vi "Instructor Write Client.vi"() -> ()   [LabVIEW 2017]
uses:
  <vilib>/OPCUA/controls/Write Status.ctl
  <vilib>/OPCUA/controls/NodeId.ctl
  <vilib>/OPCUA/client/Multiple Write Double Array.vi
  <vilib>/OPCUA/client/Multiple Write Bool Array.vi
  <vilib>/OPCUA/NI OPC UA Client.lvlib
panel:
  in  "Node Status 2":T1 items=["Good"=0, "Uncertain_InitialValue"=1083310080, "Uncertain_LastUsableValue"=1083179008, "Uncertain_SensorNotAccurate"=1083375616, "Uncertain_EngineeringUnitsExceeded"=1083441152, "Bad_NoCommunication"=2150694912, "Bad_NotReadable"=2151284736, "Bad_NotWritable"=2151350272, "Bad_OutOfRange"=2151415808, "Bad_WaitingForInitialData"=2150760448]
  in  "Time Stamp 2":timestamp
  in  "Node Status":T1 items=["Good"=0, "Uncertain_InitialValue"=1083310080, "Uncertain_LastUsableValue"=1083179008, "Uncertain_SensorNotAccurate"=1083375616, "Uncertain_EngineeringUnitsExceeded"=1083441152, "Bad_NoCommunication"=2150694912, "Bad_NotReadable"=2151284736, "Bad_NotWritable"=2151350272, "Bad_OutOfRange"=2151415808, "Bad_WaitingForInitialData"=2150760448]
  in  "Time Stamp":timestamp
  in  "Stop Broadcasting":bool
  in  "Time Stamp":timestamp
  in  "Node Status":T1 items=["Good"=0, "Uncertain_InitialValue"=1083310080, "Uncertain_LastUsableValue"=1083179008, "Uncertain_SensorNotAccurate"=1083375616, "Uncertain_EngineeringUnitsExceeded"=1083441152, "Bad_NoCommunication"=2150694912, "Bad_NotReadable"=2151284736, "Bad_NotWritable"=2151350272, "Bad_OutOfRange"=2151415808, "Bad_WaitingForInitialData"=2150760448]
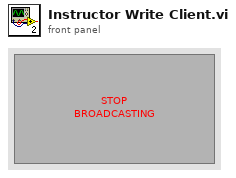
[diagram p1: front panel]
types:
  T1 = typedef "Write Status.ctl" = u32
  T2 = cluster{"message mode":enum16{"None", "Sign", "Sign and Encrypt"}, "security":enum16{"Basic256", "Basic128Rsa15"}}
  T3 = typedef "OPC UA Client Refnum.ctl" = refnum<k21>
  T4 = typedef "NodeId.ctl" = string
  T5 = cluster{"node ID":T4, "value":bool[], "timestamp (current time)":timestamp, "node status":T1}
  T6 = cluster{"node ID":T4, "value":dbl[], "timestamp (current time)":timestamp, "node status":T1}
  T7 = cluster{"node ID":T4, "value":dbl[], "timestamp (current time)":timestamp, "node status":T1}[]
  T8 = cluster{"node ID":T4, "value":bool[], "timestamp (current time)":timestamp, "node status":T1}[]
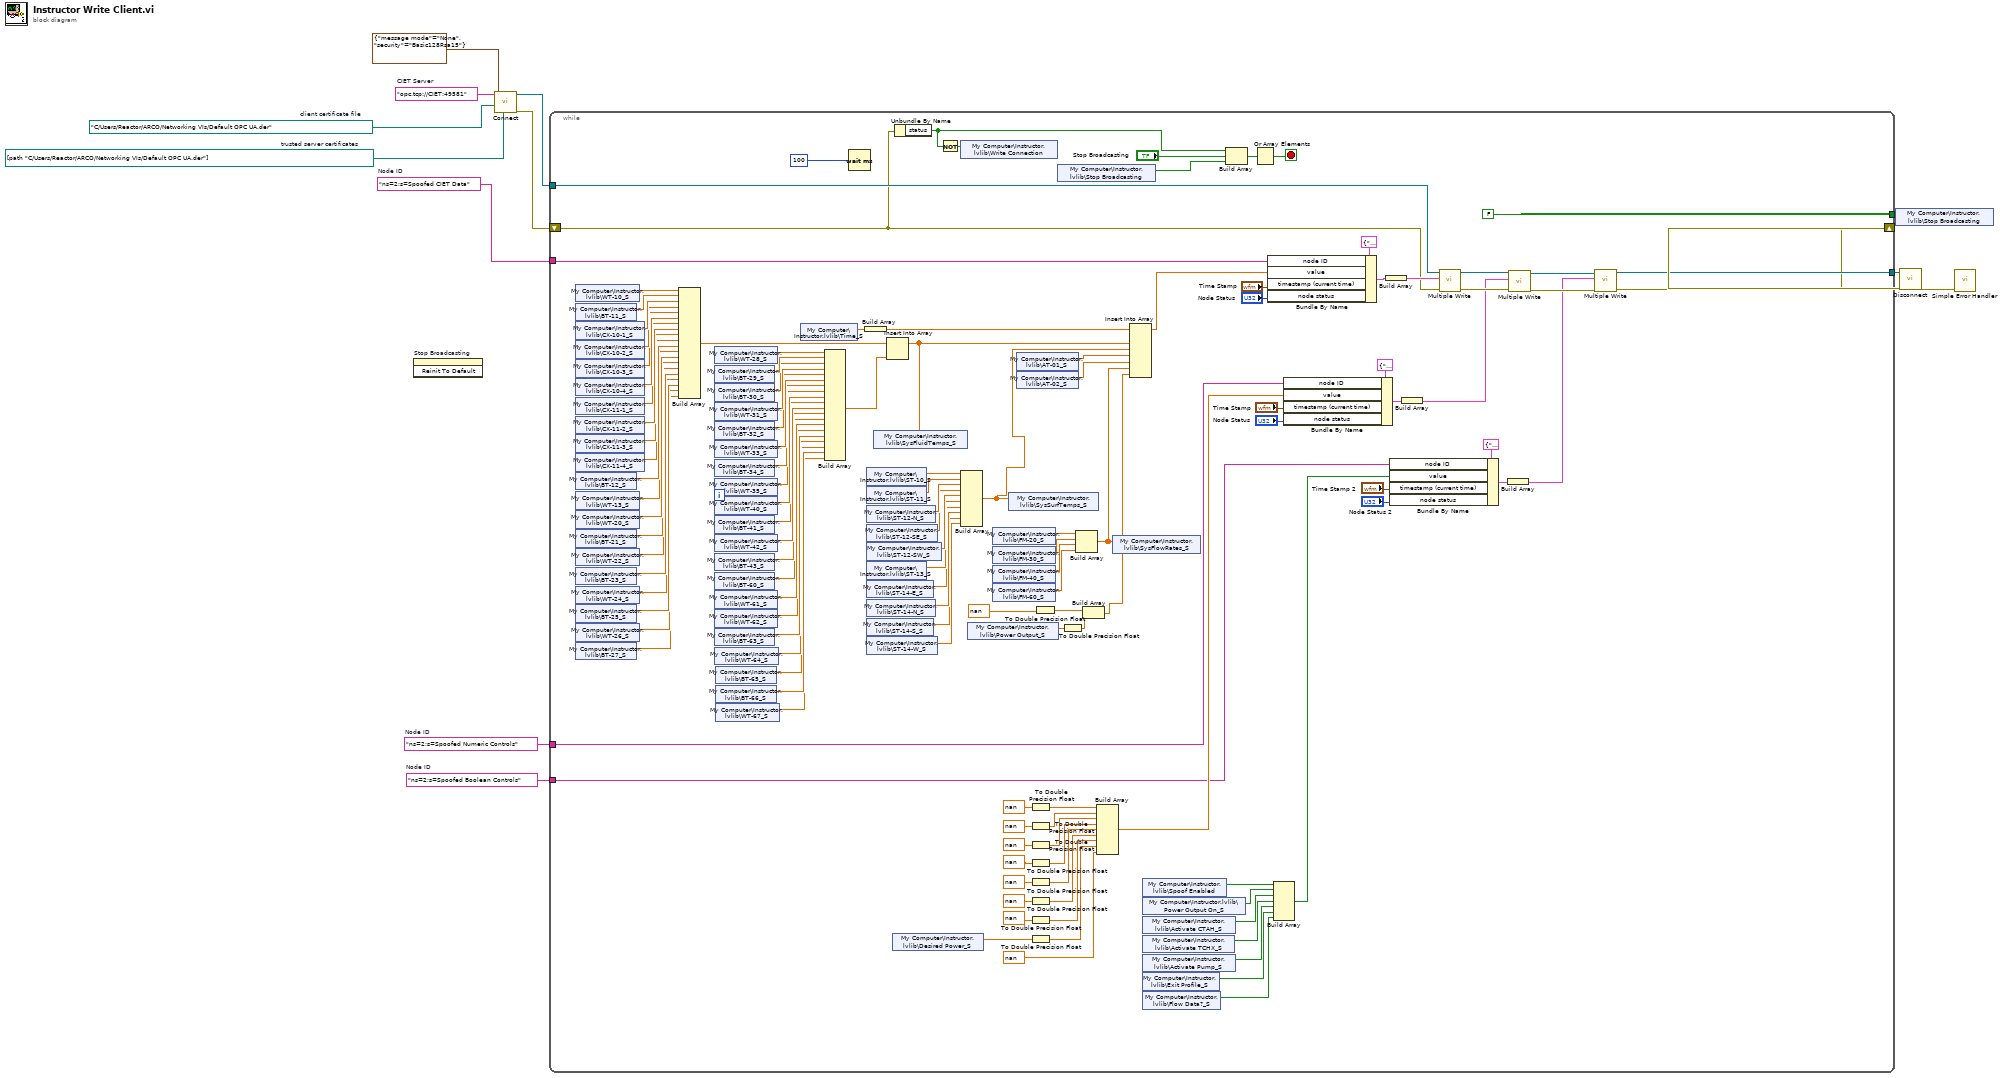
[diagram p0: block diagram]
diagram:
  w1 = "ns=2;s=Spoofed Boolean Controls"  # Node ID
  w3 = "ns=2;s=Spoofed Numeric Controls"  # Node ID
  w8 = path[] [path "C:/Users/Reactor/ARCO/Networking VIs/Default OPC UA.der"]  # trusted server certificates
  w9 = path "C:/Users/Reactor/ARCO/Networking VIs/Default OPC UA.der"  # client certificate file
  w10 = "ns=2;s=Spoofed CIET Data"  # Node ID
  w12 = "opc.tcp://CIET:49581"  # CIET Server
  n1 = invoke on="Stop Broadcasting" class="Bool (strict)" method="Reinit To Default"() -> ()  [unwired: 3 in, 3 out]
  n2 = call <vilib>:"Connect.vi"("trusted server certificates"=w8, "client certificate file"=w9, "security policy"=T2 {"message mode"=enum."None", "security"=enum."Basic128Rsa15"}, "server endpoint URL"=w12) -> ("error out"=w5:errorcluster, "OPC UA client refnum out"=w11:T3)  [unwired: 5 in, 1 out]
  n3 = while {
    tunnel: w10 -> [w141]
    tunnel: w11 -> [w140]
    tunnel: [FALSE] -> w6
    shift-right: [w29] -> w4
    shift-left: w5 -> [w63]
    tunnel: w3 -> [w57]
    tunnel: [w30] -> w2
    tunnel: w1 -> [w28]
    stop <- w69 stop-if-true
    n4 = shared-variable "My Computer\\Instructor.lvlib\\WT-10_S"() -> (w134:sgl)  [unwired: 1 in, 1 out]
    n5 = shared-variable "My Computer\\Instructor.lvlib\\BT-11_S"() -> (w133:sgl)  [unwired: 1 in, 1 out]
    n6 = shared-variable "My Computer\\Instructor.lvlib\\CX-10-1_S"() -> (w132:sgl)  [unwired: 1 in, 1 out]
    n7 = shared-variable "My Computer\\Instructor.lvlib\\CX-10-2_S"() -> (w131:sgl)  [unwired: 1 in, 1 out]
    n8 = shared-variable "My Computer\\Instructor.lvlib\\CX-10-3_S"() -> (w130:sgl)  [unwired: 1 in, 1 out]
    n9 = shared-variable "My Computer\\Instructor.lvlib\\CX-10-4_S"() -> (w129:sgl)  [unwired: 1 in, 1 out]
    n10 = shared-variable "My Computer\\Instructor.lvlib\\CX-11-1_S"() -> (w128:sgl)  [unwired: 1 in, 1 out]
    n11 = shared-variable "My Computer\\Instructor.lvlib\\CX-11-2_S"() -> (w127:sgl)  [unwired: 1 in, 1 out]
    n12 = shared-variable "My Computer\\Instructor.lvlib\\CX-11-3_S"() -> (w126:sgl)  [unwired: 1 in, 1 out]
    n13 = shared-variable "My Computer\\Instructor.lvlib\\CX-11-4_S"() -> (w125:sgl)  [unwired: 1 in, 1 out]
    n14 = shared-variable "My Computer\\Instructor.lvlib\\BT-12_S"() -> (w124:sgl)  [unwired: 1 in, 1 out]
    n15 = shared-variable "My Computer\\Instructor.lvlib\\WT-13_S"() -> (w123:sgl)  [unwired: 1 in, 1 out]
    n16 = shared-variable "My Computer\\Instructor.lvlib\\WT-20_S"() -> (w122:sgl)  [unwired: 1 in, 1 out]
    n17 = shared-variable "My Computer\\Instructor.lvlib\\BT-21_S"() -> (w121:sgl)  [unwired: 1 in, 1 out]
    n18 = shared-variable "My Computer\\Instructor.lvlib\\WT-22_S"() -> (w120:sgl)  [unwired: 1 in, 1 out]
    n19 = shared-variable "My Computer\\Instructor.lvlib\\BT-23_S"() -> (w119:sgl)  [unwired: 1 in, 1 out]
    n20 = shared-variable "My Computer\\Instructor.lvlib\\WT-24_S"() -> (w118:sgl)  [unwired: 1 in, 1 out]
    n21 = shared-variable "My Computer\\Instructor.lvlib\\BT-25_S"() -> (w117:sgl)  [unwired: 1 in, 1 out]
    n22 = shared-variable "My Computer\\Instructor.lvlib\\WT-26_S"() -> (w116:sgl)  [unwired: 1 in, 1 out]
    n23 = shared-variable "My Computer\\Instructor.lvlib\\BT-27_S"() -> (w115:sgl)  [unwired: 1 in, 1 out]
    n24 = Build Array(w134, w133, w132, w131, w130, w129, w128, w127, w126, w125, w124, w123, w122, w121, w120, w119, w118, w117, w116, w115) -> (w93:sgl[])
    n25 = shared-variable "My Computer\\Instructor.lvlib\\WT-28_S"() -> (w114:sgl)  [unwired: 1 in, 1 out]
    n26 = shared-variable "My Computer\\Instructor.lvlib\\BT-29_S"() -> (w113:sgl)  [unwired: 1 in, 1 out]
    n27 = shared-variable "My Computer\\Instructor.lvlib\\BT-30_S"() -> (w112:sgl)  [unwired: 1 in, 1 out]
    n28 = shared-variable "My Computer\\Instructor.lvlib\\WT-31_S"() -> (w111:sgl)  [unwired: 1 in, 1 out]
    n29 = shared-variable "My Computer\\Instructor.lvlib\\BT-32_S"() -> (w110:sgl)  [unwired: 1 in, 1 out]
    n30 = shared-variable "My Computer\\Instructor.lvlib\\WT-33_S"() -> (w109:sgl)  [unwired: 1 in, 1 out]
    n31 = shared-variable "My Computer\\Instructor.lvlib\\BT-34_S"() -> (w108:sgl)  [unwired: 1 in, 1 out]
    n32 = shared-variable "My Computer\\Instructor.lvlib\\WT-35_S"() -> (w107:sgl)  [unwired: 1 in, 1 out]
    n33 = shared-variable "My Computer\\Instructor.lvlib\\WT-40_S"() -> (w106:sgl)  [unwired: 1 in, 1 out]
    n34 = shared-variable "My Computer\\Instructor.lvlib\\BT-41_S"() -> (w105:sgl)  [unwired: 1 in, 1 out]
    n35 = shared-variable "My Computer\\Instructor.lvlib\\WT-42_S"() -> (w104:sgl)  [unwired: 1 in, 1 out]
    n36 = shared-variable "My Computer\\Instructor.lvlib\\BT-43_S"() -> (w103:sgl)  [unwired: 1 in, 1 out]
    n37 = shared-variable "My Computer\\Instructor.lvlib\\BT-60_S"() -> (w102:sgl)  [unwired: 1 in, 1 out]
    n38 = shared-variable "My Computer\\Instructor.lvlib\\WT-61_S"() -> (w101:sgl)  [unwired: 1 in, 1 out]
    n39 = shared-variable "My Computer\\Instructor.lvlib\\WT-62_S"() -> (w100:sgl)  [unwired: 1 in, 1 out]
    n40 = shared-variable "My Computer\\Instructor.lvlib\\BT-63_S"() -> (w99:sgl)  [unwired: 1 in, 1 out]
    n41 = shared-variable "My Computer\\Instructor.lvlib\\WT-64_S"() -> (w98:sgl)  [unwired: 1 in, 1 out]
    n42 = shared-variable "My Computer\\Instructor.lvlib\\BT-65_S"() -> (w97:sgl)  [unwired: 1 in, 1 out]
    n43 = shared-variable "My Computer\\Instructor.lvlib\\BT-66_S"() -> (w96:sgl)  [unwired: 1 in, 1 out]
    n44 = shared-variable "My Computer\\Instructor.lvlib\\WT-67_S"() -> (w95:sgl)  [unwired: 1 in, 1 out]
    n45 = shared-variable "My Computer\\Instructor.lvlib\\Time_S"() -> (w82:sgl)  [unwired: 1 in, 1 out]
    n46 = Build Array(w114, w113, w112, w111, w110, w109, w108, w107, w106, w105, w104, w103, w102, w101, w100, w99, w98, w97, w96, w95) -> (w94:sgl[])
    n47 = Wait (ms)(milliseconds to wait=u32 100) -> ()  [unwired: 1 out]
    n48 = Build Array(w82) -> (w73:sgl[])
    n49 = shared-variable "My Computer\\Instructor.lvlib\\ST-10_S"() -> (w92:sgl)  [unwired: 1 in, 1 out]
    n50 = shared-variable "My Computer\\Instructor.lvlib\\ST-11_S"() -> (w91:sgl)  [unwired: 1 in, 1 out]
    n51 = shared-variable "My Computer\\Instructor.lvlib\\ST-12-N_S"() -> (w90:sgl)  [unwired: 1 in, 1 out]
    n52 = shared-variable "My Computer\\Instructor.lvlib\\ST-12-SE_S"() -> (w89:sgl)  [unwired: 1 in, 1 out]
    n53 = shared-variable "My Computer\\Instructor.lvlib\\ST-12-SW_S"() -> (w88:sgl)  [unwired: 1 in, 1 out]
    n54 = shared-variable "My Computer\\Instructor.lvlib\\ST-13_S"() -> (w87:sgl)  [unwired: 1 in, 1 out]
    n55 = shared-variable "My Computer\\Instructor.lvlib\\ST-14-E_S"() -> (w86:sgl)  [unwired: 1 in, 1 out]
    n56 = shared-variable "My Computer\\Instructor.lvlib\\ST-14-N_S"() -> (w85:sgl)  [unwired: 1 in, 1 out]
    n57 = shared-variable "My Computer\\Instructor.lvlib\\ST-14-S_S"() -> (w84:sgl)  [unwired: 1 in, 1 out]
    n58 = shared-variable "My Computer\\Instructor.lvlib\\ST-14-W_S"() -> (w83:sgl)  [unwired: 1 in, 1 out]
    n59 = Insert Into Array(array=w93, new element=w94) -> (w81:sgl[])  [unwired: 1 in]
    n60 = shared-variable "My Computer\\Instructor.lvlib\\SysFluidTemps_S"(w81) -> ()  [unwired: 1 in, 1 out]
    n61 = shared-variable "My Computer\\Instructor.lvlib\\Desired Power_S"() -> (w50:sgl)  [unwired: 1 in, 1 out]
    n62 = Unbundle By Name(w63) -> ("status"=w65:bool)
    n63 = Not(x=w65) -> (.not. x?=w64:bool)
    n64 = shared-variable "My Computer\\Instructor.lvlib\\Write Connection"(w64) -> ()  [unwired: 1 in, 1 out]
    n65 = Build Array(w92, w91, w90, w89, w88, w87, w86, w85, w84, w83) -> (w72:sgl[])
    n66 = shared-variable "My Computer\\Instructor.lvlib\\Power Output_S"() -> (w17:sgl)  [unwired: 1 in, 1 out]
    n67 = shared-variable "My Computer\\Instructor.lvlib\\FM-20_S"() -> (w78:sgl)  [unwired: 1 in, 1 out]
    n68 = shared-variable "My Computer\\Instructor.lvlib\\FM-30_S"() -> (w77:sgl)  [unwired: 1 in, 1 out]
    n69 = shared-variable "My Computer\\Instructor.lvlib\\FM-40_S"() -> (w76:sgl)  [unwired: 1 in, 1 out]
    n70 = shared-variable "My Computer\\Instructor.lvlib\\FM-60_S"() -> (w75:sgl)  [unwired: 1 in, 1 out]
    n71 = shared-variable "My Computer\\Instructor.lvlib\\SysSurfTemps_S"(w72) -> ()  [unwired: 1 in, 1 out]
    n72 = shared-variable "My Computer\\Instructor.lvlib\\AT-01_S"() -> (w80:sgl)  [unwired: 1 in, 1 out]
    n73 = shared-variable "My Computer\\Instructor.lvlib\\AT-02_S"() -> (w79:sgl)  [unwired: 1 in, 1 out]
    n74 = To Double Precision Float(number=nan) -> (double precision float=w54:dbl)
    n75 = To Double Precision Float(number=nan) -> (double precision float=w53:dbl)
    n76 = To Double Precision Float(number=nan) -> (double precision float=w52:dbl)
    n77 = To Double Precision Float(number=nan) -> (double precision float=w51:dbl)
    n78 = To Double Precision Float(number=nan) -> (double precision float=w49:dbl)
    n79 = To Double Precision Float(number=nan) -> (double precision float=w48:dbl)
    n80 = To Double Precision Float(number=nan) -> (double precision float=w47:dbl)
    n81 = To Double Precision Float(number=w50) -> (double precision float=w46:dbl)
    n82 = To Double Precision Float(number=nan) -> (double precision float=w16:dbl)
    n83 = shared-variable "My Computer\\Instructor.lvlib\\Stop Broadcasting"() -> (w67:bool)  [unwired: 1 in, 1 out]
    n84 = To Double Precision Float(number=w17) -> (double precision float=w15:dbl)
    n85 = Build Array(w78, w77, w76, w75) -> (w74:sgl[])
    n86 = Build Array(w16, w15) -> (w14:dbl[])
    n87 = Build Array(w54, w53, w52, w51, w49, w48, w47, w46, nan ("number")) -> (w45:dbl[])
    n88 = shared-variable "My Computer\\Instructor.lvlib\\SysFlowRates_S"(w74) -> ()  [unwired: 1 in, 1 out]
    n89 = Insert Into Array(array=w73, new element #1=w81, new element #2=w72, new element #3=w80, new element #4=w79, new element #5=w74, new element #6=w14) -> (w71:sgl[])  [unwired: 1 in]
    n90 = shared-variable "My Computer\\Instructor.lvlib\\Spoof Enabled"() -> (w26:bool)  [unwired: 1 in, 1 out]
    n91 = shared-variable "My Computer\\Instructor.lvlib\\Power Output On_S"() -> (w25:bool)  [unwired: 1 in, 1 out]
    n92 = shared-variable "My Computer\\Instructor.lvlib\\Activate CTAH_S"() -> (w24:bool)  [unwired: 1 in, 1 out]
    n93 = shared-variable "My Computer\\Instructor.lvlib\\Activate TCHX_S"() -> (w23:bool)  [unwired: 1 in, 1 out]
    n94 = shared-variable "My Computer\\Instructor.lvlib\\Activate Pump_S"() -> (w22:bool)  [unwired: 1 in, 1 out]
    n95 = shared-variable "My Computer\\Instructor.lvlib\\Exit Profile_S"() -> (w21:bool)  [unwired: 1 in, 1 out]
    n96 = shared-variable "My Computer\\Instructor.lvlib\\Flow Data?_S"() -> (w20:bool)  [unwired: 1 in, 1 out]
    n97 = Build Array(w65, "Stop Broadcasting", w67) -> (w68:bool[])
    n98 = Or Array Elements(Boolean array=w68) -> (logical OR=w69:bool)
    n99 = Bundle By Name(cluster=T6 {"node ID"="", "value"=[], "timestamp (current time)"=timestamp(0 s since 1904-01-01), "node status"=0} ("request"), "node ID"=w141, "value"=w71, "timestamp (current time)"="Time Stamp", "node status"="Node Status") -> (w136:T6)
    n100 = Build Array(w26, w25, w24, w23, w22, w21, w20) -> (w27:bool[])
    n101 = Bundle By Name(cluster=T6 {"node ID"="", "value"=[], "timestamp (current time)"=timestamp(0 s since 1904-01-01), "node status"=0} ("request"), "node ID"=w57, "value"=w45, "timestamp (current time)"="Time Stamp", "node status"="Node Status") -> (w60:T6)
    n102 = Build Array(w136) -> (w135:T7)
    n103 = Bundle By Name(cluster=T5 {"node ID"="", "value"=[], "timestamp (current time)"=timestamp(0 s since 1904-01-01), "node status"=0} ("request"), "node ID"=w28, "value"=w27, "timestamp (current time)"="Time Stamp 2", "node status"="Node Status 2") -> (w36:T5)
    n104 = Build Array(w60) -> (w59:T7)
    n105 = call-poly <vilib>:"Multiple Write.vi"("error in (no error)"=w63, "requests"=w135, "OPC UA client refnum in"=w140) -> ("error out"=w61:errorcluster, "OPC UA client refnum out"=w62:T3)  [unwired: 5 in, 2 out]
    n106 = Build Array(w36) -> (w19:T8)
    n107 = call-poly <vilib>:"Multiple Write.vi"("error in (no error)"=w61, "requests"=w59, "OPC UA client refnum in"=w62) -> ("error out"=w31:errorcluster, "OPC UA client refnum out"=w32:T3)  [unwired: 5 in, 2 out]
    n108 = call-poly <vilib>:"Multiple Write.vi"("error in (no error)"=w31, "requests"=w19, "OPC UA client refnum in"=w32) -> ("error out"=w29:errorcluster, "OPC UA client refnum out"=w30:T3)  [unwired: 5 in, 2 out]
  }
  n109 = shared-variable "My Computer\\Instructor.lvlib\\Stop Broadcasting"(w6) -> ()  [unwired: 1 in, 1 out]
  n110 = call <vilib>:"Disconnect.vi"("error in (no error)"=w4, "OPC UA client refnum in"=w2) -> ("error out"=w13:errorcluster)  [unwired: 9 in]
  n111 = call <vilib>:"Simple Error Handler.vi"("error in (no error)"=w13) -> ()  [unwired: 4 in, 5 out]
